vi "Daqmx analog read.vi"(8 "Focus or flystart?":bool, 9 "error in":errorcluster, 10 "task in":refnum<k21>, 11 "Timeout (s)":dbl) -> (0 "error out":errorcluster, 1 "DAQ loop terminated?":bool, 2 "queue out":refnum<queue>, 3 "task out":refnum<k21>)   [LabVIEW 2017]
uses:
  <vilib>/DAQmx/read.llb/DAQmx Read (Analog 2D I16 NChan NSamp).vi
  GFG/GFGbooleanGet.vi
  GFG/GFGnumericGet.vi
  <vilib>/DAQmx/miscellaneous.llb/DAQmx Fill In Error Info.vi
  GFG/GFG library.lvlib
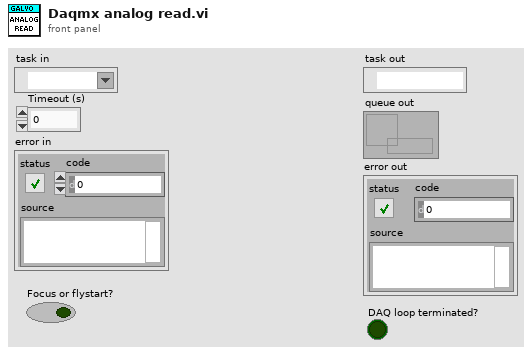
[diagram p1: front panel]
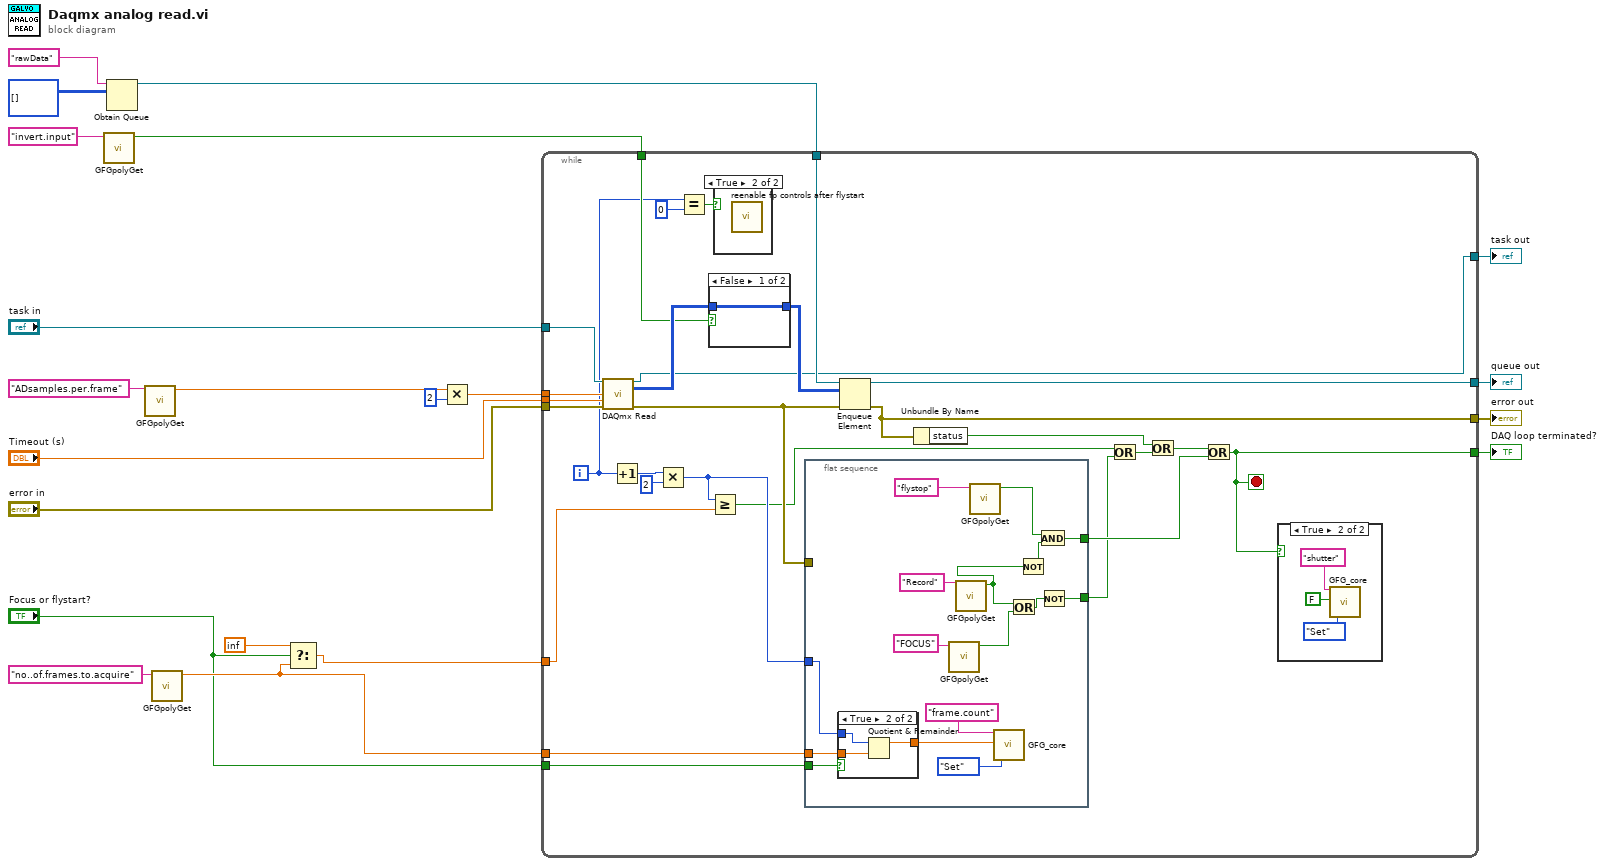
[diagram p0: block diagram]
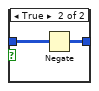
[diagram p3: hidden frame]
diagram:
  n1 = call-poly "GFGpolyGet.vi"("Variable Name in"="invert.input" ("Tag in")) -> ("Boolean Value OUT"=w17:bool)  [unwired: 9 in, 1 out]
  n2 = Obtain Queue(name (unnamed)="rawData", element data type=i16[][] [] ("-x")) -> (queue out=w19:refnum<queue>)  [unwired: 3 in, 2 out]
  n3 = call-poly "GFGpolyGet.vi"("Variable Name in"="ADsamples.per.frame" ("Tag in")) -> ("Numeric"=w13:dbl)  [unwired: 8 in, 2 out]
  n4 = call-poly "GFGpolyGet.vi"("Variable Name in"="no..of.frames.to.acquire" ("Tag in")) -> ("Numeric"=w6:dbl)  [unwired: 8 in, 2 out]
  n5 = Select(t=inf, s="Focus or flystart?", f=w6) -> (s? t:f=w7:dbl)
  n6 = Multiply(x=w13, y=i8 2) -> (x*y=w12:dbl)
  n7 = while {
    tunnel: [w43] -> w4
    tunnel: [w42] -> w2
    tunnel: w12 -> [w45]
    tunnel: w19 -> [w48]
    tunnel: [w47] -> w3
    tunnel: w7 -> [w44]
    tunnel: "Timeout (s)" -> [w41]
    tunnel: "error in" -> [w37]
    tunnel: w17 -> [w36]
    tunnel: "task in" -> [w34]
    tunnel: "Focus or flystart?" -> [w30]
    tunnel: w6 -> [w29]
    tunnel: [w26] -> w1
    i -> [w23]
    stop <- w26 stop-if-true
    n8 = call-poly <vilib>:"DAQmx Read.vi"("task/channels in"=w34, "number of samples per channel"=w45, "timeout"=w41, "error in"=w37) -> ("task out"=w43:refnum<k21>, "data"=w46:i16[][], "error out"=w38:errorcluster)  [unwired: 9 in]
    n9 = Increment(x=w23) -> (x+1=w40:i32)
    n10 = Multiply(x=w40, y=2) -> (x*y=w35:i32)
    n11 = Equal?(x=w23, y=0) -> (x = y?=w24:bool)
    n12 = case shown="False" w36 {
      tunnel: [w50 w52] -> w49
      tunnel: w46 -> [w50 w51]
      frame False {
      }
      frame True {
        n13 = Negate(x=w51) -> (-x=w52:i16[][])
      }
    }
    n14 = Greater Or Equal?(x=w35, y=w44) -> (x >= y?=w32:bool)
    n15 = case shown="True" w24 {
      frame False {
      }
      frame True {
        n16 = call "reenable fp controls after flystart.vi"() -> ()  [unwired: 12 in]
      }
    }
    n17 = flat-sequence {
      tunnel: w38 -> [_]
      tunnel: w35 -> [w62]
      tunnel: w30 -> [w65]
      tunnel: w29 -> [w63]
      tunnel: [w57] -> w27
      tunnel: [w55] -> w25
      frame #0 {
        n18 = case shown="True" w65 {
          tunnel: w63 -> [_ w72]
          tunnel: w62 -> [w69 w71]
          tunnel: [w69 w70] -> w61
          frame False {
          }
          frame True {
            n19 = Quotient & Remainder(x=w71, y=w72) -> (x-y*floor(x/y)=w70:dbl)  [unwired: 1 out]
          }
        }
        n20 = call-poly "GFGpolyGet.vi"("Variable Name in"="FOCUS") -> ("Boolean Value OUT"=w53:bool)  [unwired: 9 in, 1 out]
        n21 = call-poly "GFGpolyGet.vi"("Variable Name in"="Record") -> ("Boolean Value OUT"=w54:bool)  [unwired: 9 in, 1 out]
        n22 = call-poly "GFGpolyGet.vi"("Variable Name in"="flystop") -> ("Boolean Value OUT"=w58:bool)  [unwired: 9 in, 1 out]
        n23 = call "GFG_core.vi"("Variable Name in"="frame.count", "Variant in"=w61, "Action"=enum16{"Init", "Set", "Get"}."Set") -> ()  [unwired: 10 in, 7 out]
        n24 = Or(x=w54, y=w53) -> (x .or. y?=w56:bool)
        n25 = Not(x=w54) -> (.not. x?=w59:bool)
        n26 = And(x=w58, y=w59) -> (x .and. y?=w57:bool)
        n27 = Not(x=w56) -> (.not. x?=w55:bool)
      }
    }
    n28 = Enqueue Element(queue=w48, element=w49, error in (no error)=w38) -> (queue out=w47:refnum<queue>, error out=w42:errorcluster)  [unwired: 1 in, 1 out]
    n29 = Unbundle By Name(w42) -> ("status"=w33:bool)
    n30 = Or(x=w32, y=w25) -> (x .or. y?=w31:bool)
    n31 = Or(x=w33, y=w31) -> (x .or. y?=w28:bool)
    n32 = Or(x=w28, y=w27) -> (x .or. y?=w26:bool)
    n33 = case shown="True" w26 {
      frame False {
      }
      frame True {
        n34 = call "GFG_core.vi"("Variable Name in"="shutter" ("Tag in"), "Variant in"=FALSE ("Boolean"), "Action"=enum16{"Init", "Set", "Get"}."Set") -> ()  [unwired: 10 in, 7 out]
      }
    }
  }
  "task out" <- w4
  "queue out" <- w3
  "error out" <- w2
  "DAQ loop terminated?" <- w1
